vi "HW3part1.vi"() -> ()   [LabVIEW 2015]
panel:
  in  "Boolean":bool
  in  "stop":bool
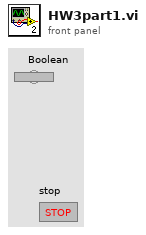
[diagram p1: front panel]
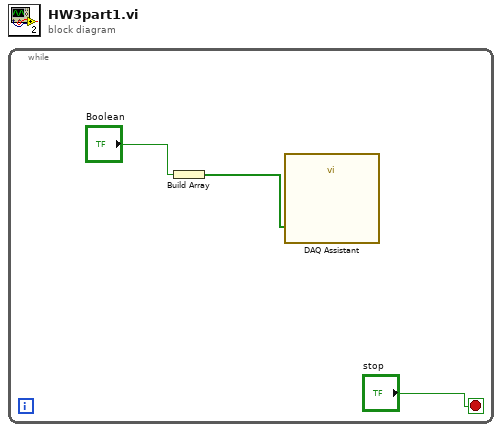
[diagram p0: block diagram]
diagram:
  n1 = while {
    stop <- "stop" stop-if-true
    n2 = Build Array("Boolean") -> (w2:bool[])
    n3 = call "DAQ Assistant"("data"=w2) -> ()  [unwired: 17 in, 2 out]
  }
